vi "contains_node.vi"(10 "Node":cluster{"Weight":dbl, "Row":dbl, "Col":dbl}, 11 "Cost_so_far":T1(array[cluster])) -> (3 "output":bool)   [LabVIEW 2014]
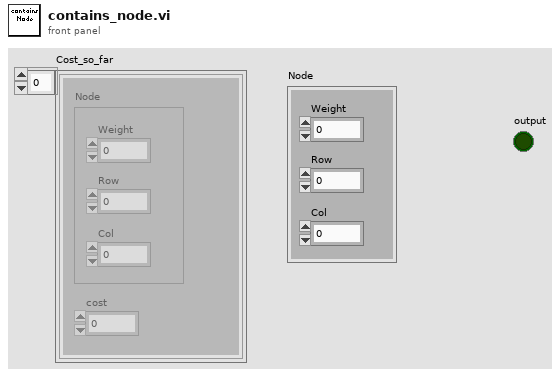
[diagram p1: front panel]
types:
  T1 = cluster{"Node":cluster{"Weight":dbl, "Row":dbl, "Col":dbl}, "cost":dbl}[]
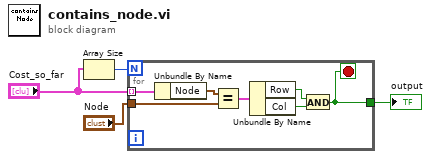
[diagram p0: block diagram]
diagram:
  n1 = Array Size(array="Cost_so_far") -> (size(s)=w4:i32)
  n2 = for {
    N: w4 -> [_]
    tunnel: "Node" -> [w9]
    tunnel: "Cost_so_far" -> [w11] mode=indexing
    tunnel: [w5] -> w1
    stop <- w5 stop-if-true
    n3 = Unbundle By Name(w11) -> ("Node"=w10:cluster{"Weight":dbl, "Row":dbl, "Col":dbl})
    n4 = Equal?(x=w10, y=w9) -> (x = y?=w8:cluster{"Weight":bool, "Row":bool, "Col":bool})
    n5 = Unbundle By Name(w8) -> ("Row"=w7:bool, "Col"=w6:bool)
    n6 = And(x=w7, y=w6) -> (x .and. y?=w5:bool)
  }
  "output" <- w1
